vi "Read Scale Props.vi"(11 "GraphScale":refnum<vi>) -> (2 "GraphScale Props":T1)   [LabVIEW 2020, in "VolatusGUIEditorCore.lvlib"]
uses:
  VolatusGUIEditorCore.lvlib
  Chart Scale Props.ctl
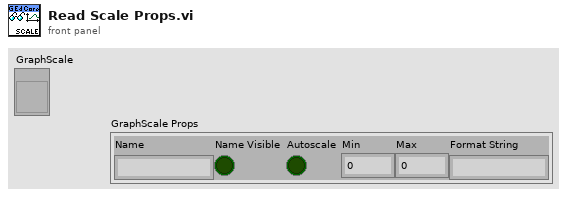
[diagram p1: front panel]
types:
  T1 = typedef "VolatusGUIEditorCore.lvlib/Chart Scale Props.ctl" = cluster{"Name":string, "Name Visible":bool, "Autoscale":bool, "Min":dbl, "Max":dbl, "Format String":string}
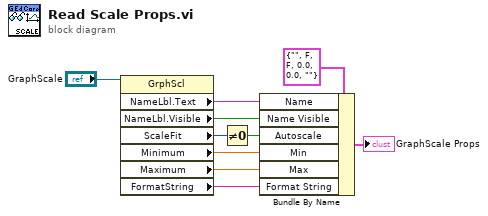
[diagram p0: block diagram]
diagram:
  n1 = property class="GrphScl"(reference="GraphScale") -> ("NameLbl.Text"=w9:string, "NameLbl.Visible"=w8:bool, "ScaleFit"=w7:u8, "Minimum"=w5:dbl, "Maximum"=w4:dbl, "FormatString"=w3:string)  [unwired: 1 in, 2 out]
  n2 = Not Equal To 0?(x=w7) -> (x != 0?=w6:bool)
  n3 = Bundle By Name(cluster=T1 {"Name"="", "Name Visible"=FALSE, "Autoscale"=FALSE, "Min"=0.0, "Max"=0.0, "Format String"=""} ("Chart Scale Props"), "Name"=w9, "Name Visible"=w8, "Autoscale"=w6, "Min"=w5, "Max"=w4, "Format String"=w3) -> (→"GraphScale Props":T1)
